vi "ExpLogSave.vi"() -> ()   [LabVIEW 2019]
uses:
  controls/GlobalExp.vi
  Global.lvlib
panel:
  in  "String":string="Please select where to save the experiment log file. Default will save to \"explog_[date].txt\""
  in  "Select":bool
  in  "Default":bool
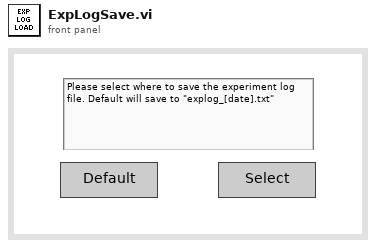
[diagram p1: front panel]
types:
  T1 = enum16{"open", "replace", "create", "open or create", "replace or create", "replace or create with confirmation"}
  T2 = typedef "MasterExpControl.ctl" = cluster{"Main Steps":dbl, "Main Runs":dbl, "ExpStatus":enum16{"Innit", "Stop", "Idle", "MainRunning", "AuxRunning"}, "Main Current Step":dbl, "ExpNum":dbl, "NewData":bool, "date":string, "command":string, "Stop":bool, "Pause":bool, "Mathematica":string, "Main/Meta":bool, "UpdateMath":bool, "Camera":bool, "MetaExpOver":bool, "NextMetaExp":bool}
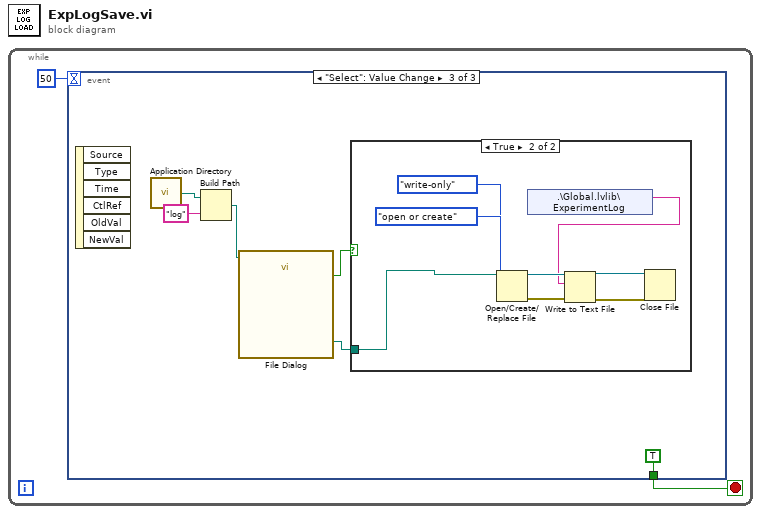
[diagram p0: block diagram]
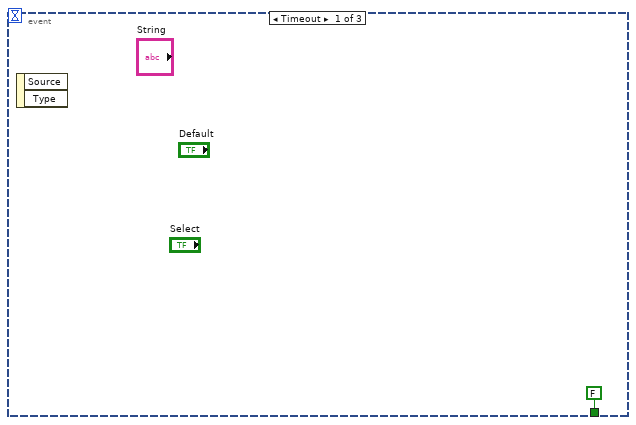
[diagram p2: hidden frame]
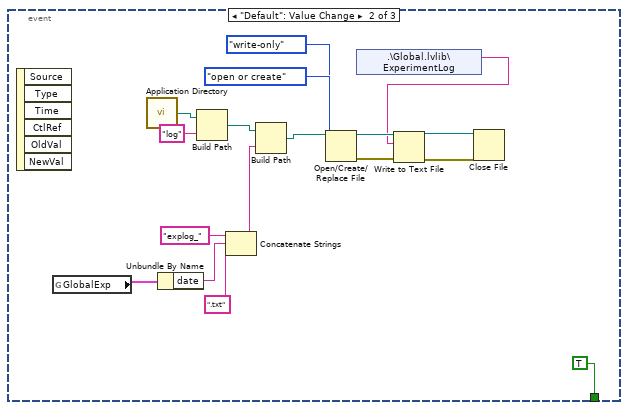
[diagram p3: hidden frame]
diagram:
  n1 = while {
    stop <- w1 stop-if-true
    n2 = event shown="[2] \"Select\": Value Change" {
      selector: _ -> [_ _ _]
      dyn-events: _ -> [_ _ _]
      timeout: 50 -> [_ _ _]
      tunnel: [FALSE TRUE TRUE] -> w1
      event Timeout {
        n3 = event-data() -> ()  [unwired: 1 in, 2 out]
      }
      event "Default": Value Change {
        n4 = event-data() -> ()  [unwired: 1 in, 6 out]
        n5 = global read "GlobalExp.vi" "GlobalExp"() -> (w17:T2)
        n6 = call <vilib>:"Application Directory.vi"() -> ("Application Directory"=w20:path)
        n7 = Unbundle By Name(w17) -> ("date"=w13:string)
        n8 = Build Path(base path=w20, name or relative path="log") -> (appended path=w18:path)
        n9 = Concatenate Strings("explog_" ("string"), w13, ".txt" ("string")) -> (w10:string)
        n10 = Build Path(base path=w18, name or relative path=w10) -> (appended path=w16:path)
        n11 = Open/Create/Replace File(file path (use dialog)=w16, operation (0:open)=T1."open or create", access (0:read/write)=enum16{"read/write", "read-only", "write-only"}."write-only") -> (refnum out=w9:refnum<file>, error out=w8:errorcluster)  [unwired: 3 in, 1 out]
        n12 = shared-variable ".\\Global.lvlib\\ExperimentLog"() -> (w5:string)  [unwired: 1 in, 1 out]
        n13 = Write to Text File(file (use dialog)=w9, text=w5, error in=w8) -> (refnum out=w7:refnum<file>, error out=w6:errorcluster)  [unwired: 1 in, 1 out]
        n14 = Close File(refnum=w7, error in=w6) -> ()  [unwired: 2 out]
      }
      event "Select": Value Change {
        n15 = event-data() -> ()  [unwired: 1 in, 6 out]
        n16 = call <vilib>:"Application Directory.vi"() -> ("Application Directory"=w26:path)
        n17 = Build Path(base path=w26, name or relative path="log") -> (appended path=w22:path)
        n18 = call "File Dialog"("start path"=w22) -> ("selected path"=w24:path, "exists"=w23:bool)  [unwired: 11 in, 2 out]
        n19 = case shown="True" w23 {
          tunnel: w24 -> [_ w27]
          frame False {
          }
          frame True {
            n20 = Open/Create/Replace File(file path (use dialog)=w27, operation (0:open)=T1."open or create", access (0:read/write)=enum16{"read/write", "read-only", "write-only"}."write-only") -> (refnum out=w32:refnum<file>, error out=w31:errorcluster)  [unwired: 3 in, 1 out]
            n21 = shared-variable ".\\Global.lvlib\\ExperimentLog"() -> (w28:string)  [unwired: 1 in, 1 out]
            n22 = Write to Text File(file (use dialog)=w32, text=w28, error in=w31) -> (refnum out=w30:refnum<file>, error out=w29:errorcluster)  [unwired: 1 in, 1 out]
            n23 = Close File(refnum=w30, error in=w29) -> ()  [unwired: 2 out]
          }
        }
      }
    }
  }
